vi "Deploy Files.vi"(8 "error in (no error)":errorcluster, 10 "Generated files":path[](array[path]), 11 "Paths in":path[](array[path])) -> (0 "error out":errorcluster)   [LabVIEW 2017]
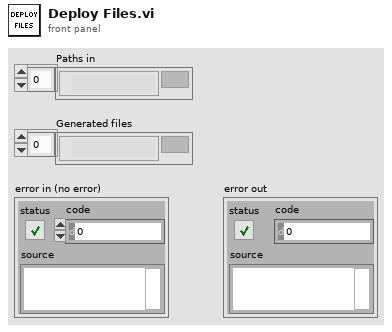
[diagram p1: front panel]
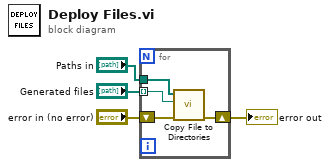
[diagram p0: block diagram]
diagram:
  n1 = for {
    tunnel: "Paths in" -> [w8]
    shift-right: [w6] -> w3
    shift-left: "error in (no error)" -> [w7]
    tunnel: "Generated files" -> [w5] mode=indexing
    n2 = call "Copy File to Directories.vi"("error in (no error)"=w7, "File to Deploy"=w5, "Paths in"=w8) -> ("error out"=w6:errorcluster)  [unwired: 7 in, 1 out]
  }
  "error out" <- w3
